vi "Initialize Error Log.vi"(8 "error in (no error)":errorcluster, 10 "Application Name":string, 11 "Logger.Error in":refnum<class "Logger.Error.lvclass">) -> (0 "error out":errorcluster, 3 "Logger.Error out":refnum<class "Logger.Error.lvclass">)   [LabVIEW 2019, in "Logger.Error.lvlib" / "Logger.Error.lvclass"]
uses:
  Logger.Error.lvclass
  <vilib>/Utility/sysdir.llb/System Directory Type.ctl
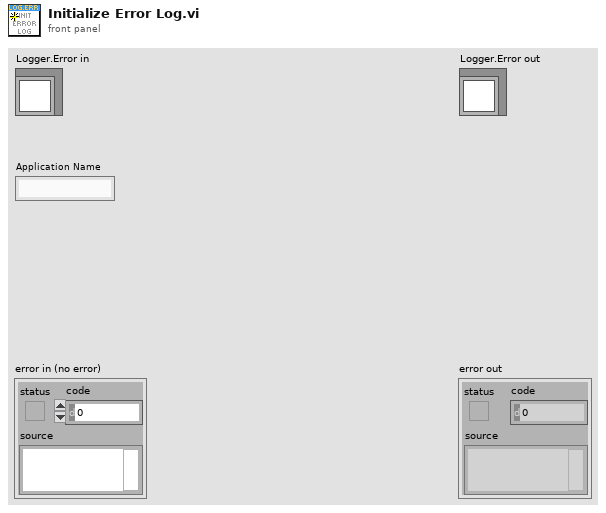
[diagram p1: front panel]
types:
  T1 = typedef "System Directory Type.ctl" = i32
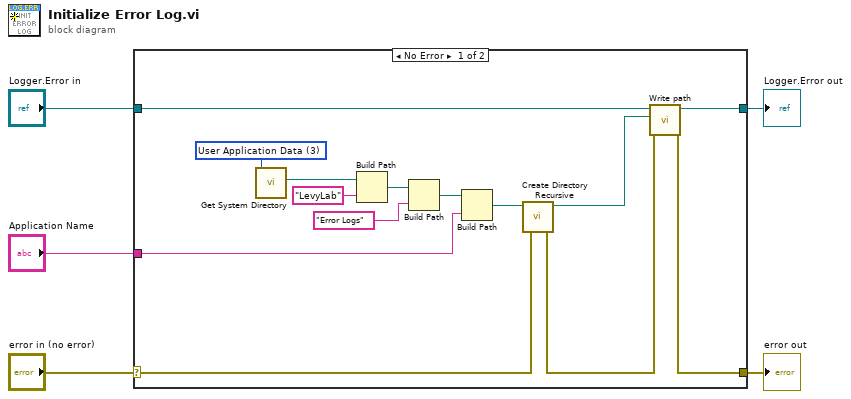
[diagram p0: block diagram]
diagram:
  n1 = case shown="No Error" "error in (no error)" {
    selector: "error in (no error)" -> [w10 w21]
    tunnel: [w6 w21] -> w4
    tunnel: [w9 w20] -> w2
    tunnel: "Logger.Error in" -> [w8 w20]
    tunnel: "Application Name" -> [w11 _]
    frame No Error {
      w17 = T1 3 items=["User Home"=0, "User Desktop"=1, "User Documents"=2, "User Application Data"=3, "User Preferences"=4, "User Temporary"=5, "Public Documents"=6, "Public Application Data"=7, "Public Preferences"=8, "Public Cache"=13, "System Core Libraries"=9, "System Installed Libraries"=10, "Application Files"=11, "Boot Volume Root"=12] ("system directory type")
      n2 = call <vilib>:"Get System Directory.vi"("system directory type"=w17) -> ("system directory"=w19:path)  [unwired: 10 in]
      n3 = Build Path(base path=w19, name or relative path="LevyLab") -> (appended path=w16:path)
      n4 = Build Path(base path=w16, name or relative path="Error Logs") -> (appended path=w14:path)
      n5 = Build Path(base path=w14, name or relative path=w11) -> (appended path=w13:path)
      n6 = call <vilib>:"Create Directory Recursive.vi"("error in (no error)"=w10, "directory"=w13) -> ("error out"=w7:errorcluster, "directory copy"=w12:path)  [unwired: 3 in, 1 out]
      n7 = call-dynamic "Write path.vi"("error in (no error)"=w7, "folder"=w12, "Logger in"=w8) -> ("error out"=w6:errorcluster, "Logger out"=w9:refnum<class "Logger.Error.lvclass">)  [unwired: 7 in]
    }
    frame Error {
    }
  }
  "error out" <- w4
  "Logger.Error out" <- w2
